vi "LSX Get TVR Out Resolution.vi"(0 "lLSID":i32, 1 "plR":i32, 5 "plX":i32, 7 "plY":i32, 9 "plZ":i32, 11 "error in (no error)":errorcluster) -> (3 "plR out":i32, 4 "function return":i32, 6 "plX out":i32, 8 "plY out":i32, 10 "plZ out":i32, 15 "error out":errorcluster)   [LabVIEW 2018, in "Tango.lvlib"]
doc: "TANGOAPI int TANGOCALL LSX_GetTVROutResolution (int lLSID, int *plX, int *plY, int *plZ, int *plR);"
uses:
  <userlib>/Tango/Tango.lvlib
  <userlib>/Tango/Tango_DLL.dll
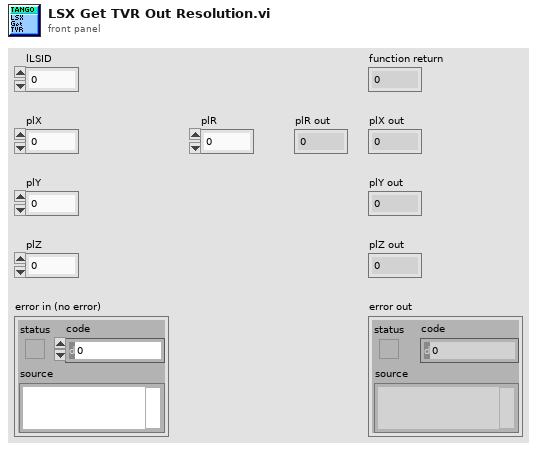
[diagram p1: front panel]
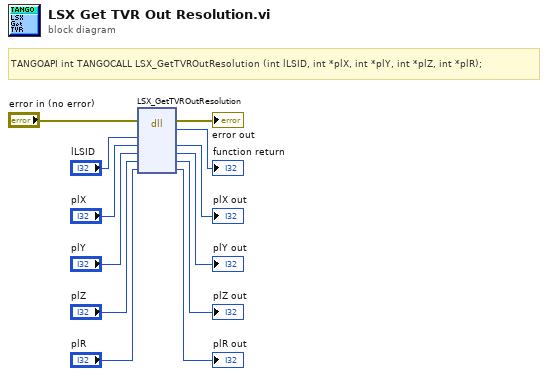
[diagram p0: block diagram]
diagram:
  # "TANGOAPI int TANGOCALL LSX_GetTVROutResolution (int lLSID, int *plX, int *plY, int *plZ, int *plR);"
  n1 = dll-call lib="C:/Program Files (x86)/National Instruments/LabVIEW 2018/user.lib/Tango/Tango_DLL.*" fn="LSX_GetTVROutResolution"(error in="error in (no error)", "lLSID"="lLSID", "plX"="plX", "plY"="plY", "plZ"="plZ", "plR"="plR") -> (error out=→"error out":errorcluster, →"function return":i32, "plX"=→"plX out":i32, "plY"=→"plY out":i32, "plZ"=→"plZ out":i32, "plR"=→"plR out":i32)  [unwired: 3 in, 1 out]
